vi "ReadHemisphereData.vi"(8 "Error in":errorcluster, 10 "Queue in":refnum<queue>, 11 "VISA UART port":refnum<visa-resource-name>) -> (0 "Error out":errorcluster)   [LabVIEW 2013]
panel:
  out "Longitude [deg]":string
  out "Latitude [deg]":string
  in  "time zone":i32
  out "Time":string
  out "Mode":string
  out "Date [ddmmyy]":string
  out "Course over ground [degrees]":string
  out "Status":string
  out "Speed over ground [knots]":string
  out "E/W":string
  out "Longitude":string
  out "N/S":string
  out "Latitude":string
  out "UTC Time":string
  out "1PPS":bool
  out "NMEA sentences":string
  # "GPS demo"
  # "[hhmmss.sss]"
  # "A = vAlid data\nV = inValid data"
  # "[ddmm.mmmm]"
  # "[dddmm.mmmm]"
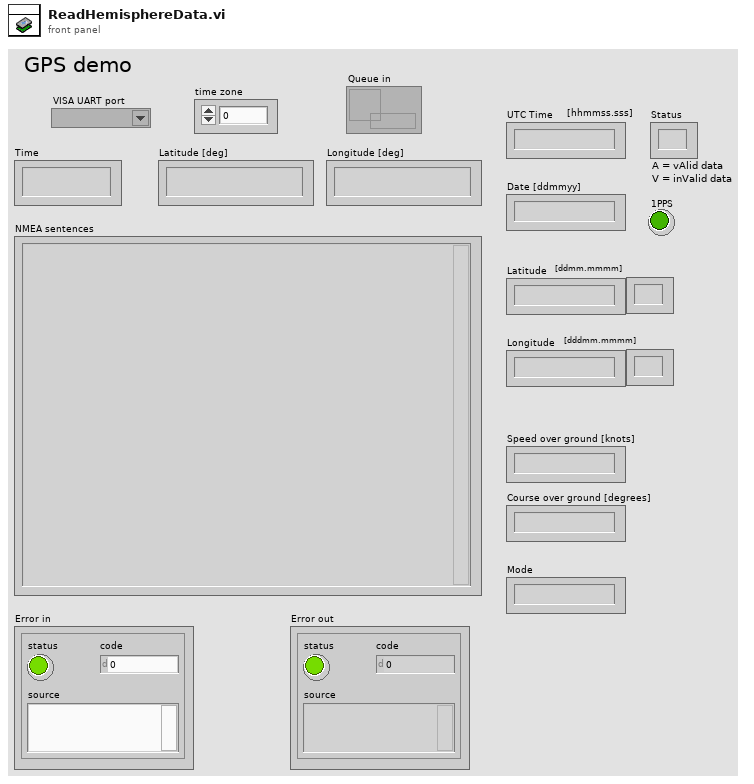
[diagram p1: front panel]
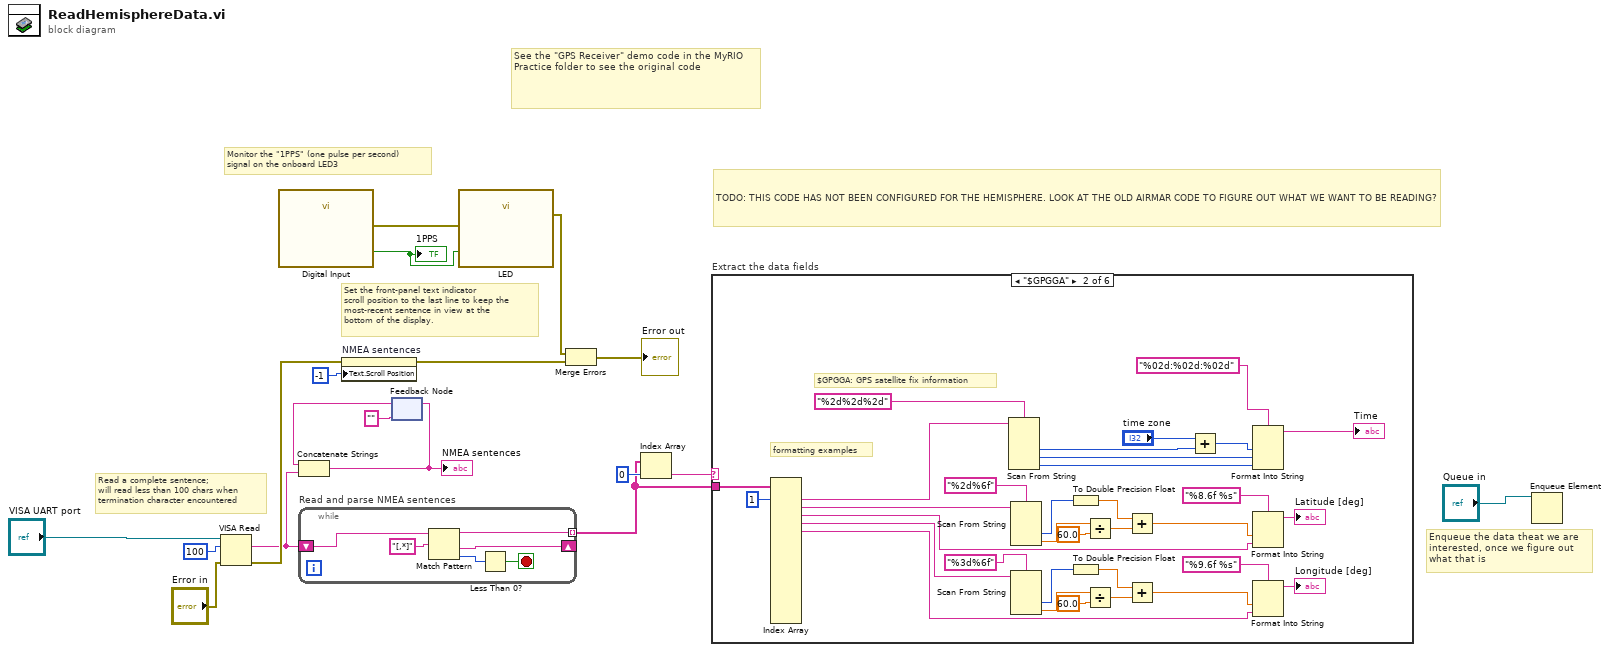
[diagram p0: block diagram]
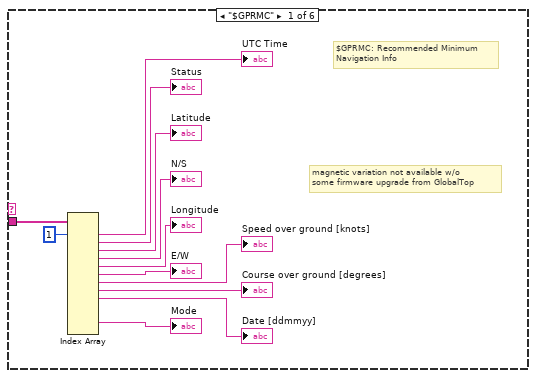
[diagram p2: hidden frame]
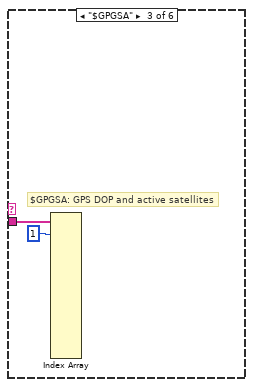
[diagram p3: hidden frame]
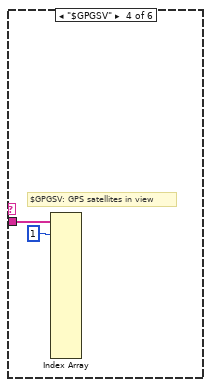
[diagram p4: hidden frame]
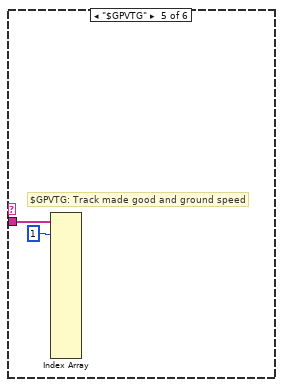
[diagram p5: hidden frame]
diagram:
  # "Enqueue the data theat we are interested, once we figure out what that is"
  # "TODO: THIS CODE HAS NOT BEEN CONFIGURED FOR THE HEMISPHERE. LOOK AT THE OLD AIRMAR CODE TO FIGURE OUT WHAT WE WANT TO BE READING?"
  # "Set the front-panel text indicator\nscroll position to the last line to keep the\nmost-recent sentence in view at the\nbottom of the display."
  # "Read a complete sentence;\nwill read less than 100 chars when\ntermination character encountered"
  # "Monitor the \"1PPS\" (one pulse per second)\nsignal on the onboard LED3"
  # "See the \"GPS Receiver\" demo code in the MyRIO Practice folder to see the original code"
  n1 = VISA Read(VISA resource name="VISA UART port", byte count=u32 100, error in (no error)="Error in") -> (read buffer=w9:string, error out=w14:errorcluster)  [unwired: 2 out]
  n2 = call "Digital Input"() -> ("A/DIO0 (Pin 11)"=w16:bool, "error out"=w17:errorcluster)  [unwired: 26 in]
  "1PPS" <- w16
  n3 = while "Read and parse NMEA sentences" {
    tunnel: [w22] -> w11 mode=indexing
    shift-right: [w21] -> _
    shift-left: w9 -> [w23]
    stop <- w20 stop-if-true
    n4 = Match Pattern(string=w23, regular expression="[,*]") -> (before substring=w22:string, after substring=w21:string, offset past match=w19:i32)  [unwired: 1 in, 1 out]
    n5 = Less Than 0?(x=w19) -> (x < 0?=w20:bool)
  }
  n6 = property on="NMEA sentences" class="Str"(error in=w14, "Text.Scroll Position"=-1) -> (error out=w2:errorcluster)  [unwired: 1 in, 1 out]
  n7 = feedback #1("") -> (w7:string)
  n8 = Concatenate Strings "Concatenate Strings"(w7, w9) -> (w5:string)
  "NMEA sentences" <- w5
  n9 = feedback-in #1(w5) -> ()
  n10 = call "LED"("LED3"=w16, "error in (no error)"=w17) -> ("error out"=w15:errorcluster)  [unwired: 25 in]
  n11 = Merge Errors "Merge Errors"(w15, w2) -> (→"Error out":errorcluster)
  n12 = Index Array "Index Array"(array=w11, index=0) -> (element=w10:string)
  n13 = case "Extract the data fields" shown="\"$GPGGA\"" w10 {
    tunnel: w11 -> [w36 w69 w71 w73 w75 _]
    frame "$GPRMC" {
      # "magnetic variation not available w/o\nsome firmware upgrade from GlobalTop"
      # "$GPRMC: Recommended Minimum\nNavigation Info"
      n14 = Index Array "Index Array"(array=w36, index #1=1 ("index")) -> (element #1=→"UTC Time":string, element #2=→"Status":string, element #3=→"Latitude":string, element #4=→"N/S":string, element #5=→"Longitude":string, element #6=→"E/W":string, element #7=→"Speed over ground [knots]":string, element #8=→"Course over ground [degrees]":string, element #9=→"Date [ddmmyy]":string, element #12=→"Mode":string)  [unwired: 12 in, 3 out]
    }
    frame "$GPGGA" {
      # "formatting examples"
      # "$GPGGA: GPS satellite fix information"
      n15 = Index Array "Index Array"(array=w69, index #1=1 ("index")) -> (element #1=w66:string, element #2=w57:string, element #3=w49:string, element #4=w38:string, element #5=w37:string)  [unwired: 15 in, 11 out]
      n16 = Scan From String "Scan From String"(format string="%2d%2d%2d", input string=w66) -> (output 1=w59:i32, output 2=w62:i32, output 3=w64:i32)  [unwired: 5 in, 3 out]
      n17 = Scan From String(format string="%2d%6f", input string=w57) -> (output 1=w54:i32, output 2=w56:dbl)  [unwired: 4 in, 3 out]
      n18 = Scan From String(format string="%3d%6f", input string=w38) -> (output 1=w42:i32, output 2=w40:dbl)  [unwired: 4 in, 3 out]
      n19 = To Double Precision Float(number=w54) -> (double precision float=w52:dbl)
      n20 = To Double Precision Float(number=w42) -> (double precision float=w44:dbl)
      n21 = Divide(x=w56, y=60.0) -> (x/y=w53:dbl)
      n22 = Divide(x=w40, y=60.0) -> (x/y=w43:dbl)
      n23 = Add(x=w52, y=w53) -> (x+y=w50:dbl)
      n24 = Add(x=w44, y=w43) -> (x+y=w46:dbl)
      n25 = Add(x="time zone", y=w59) -> (x+y=w60:i32)
      n26 = Format Into String "Format Into String"(format string="%02d:%02d:%02d", w60, w62, w64) -> (resulting string=→"Time":string)  [unwired: 2 in, 1 out]
      n27 = Format Into String(format string="%8.6f %s", w50, w49) -> (resulting string=→"Latitude [deg]":string)  [unwired: 2 in, 1 out]
      n28 = Format Into String(format string="%9.6f %s", w46, w37) -> (resulting string=→"Longitude [deg]":string)  [unwired: 2 in, 1 out]
    }
    frame "$GPGSA" {
      # "$GPGSA: GPS DOP and active satellites"
      n29 = Index Array(array=w71, index #1=1 ("index")) -> ()  [unwired: 15 in, 16 out]
    }
    frame "$GPGSV" {
      # "$GPGSV: GPS satellites in view"
      n30 = Index Array(array=w73, index #1=1 ("index")) -> ()  [unwired: 15 in, 16 out]
    }
    frame "$GPVTG" {
      # "$GPVTG: Track made good and ground speed"
      n31 = Index Array(array=w75, index #1=1 ("index")) -> ()  [unwired: 15 in, 16 out]
    }
    frame Default {
    }
  }
  n32 = Enqueue Element(queue="Queue in") -> ()  [unwired: 3 in, 3 out]
